vi "Configure slider scale.vi"(8 "error in (no error)":errorcluster, 10 "Slide Parameters":T1, 11 "Slide in":refnum<vi>) -> (0 "error out":errorcluster, 3 "Slide reference out":refnum<vi>)   [LabVIEW 2013]
uses:
  Support/Slide Parameters.ctl
  Support/PWM Object Parameters.ctl
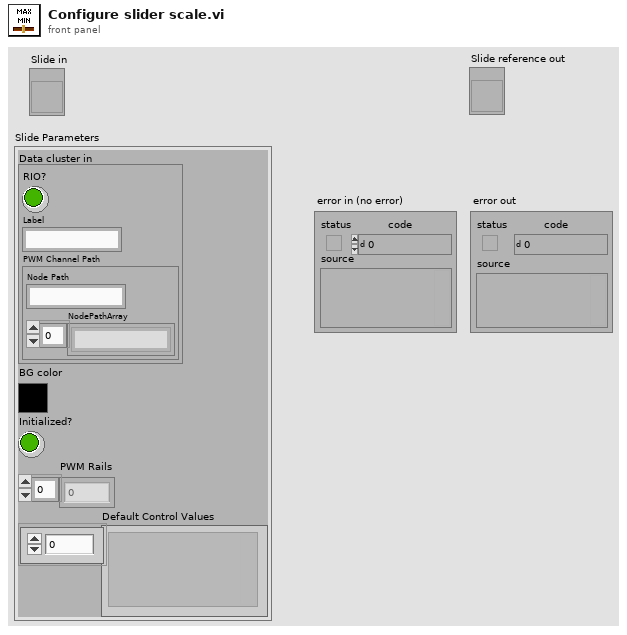
[diagram p1: front panel]
types:
  T1 = typedef "Slide Parameters.ctl" = cluster{"Data cluster in":T2, "BG color":u32, "Initialized?":bool, "PWM Rails":dbl[], "Default Control Values":variant[]}
  T2 = typedef "PWM Object Parameters.ctl" = cluster{"RIO?":bool, "Label":string, "PWM Channel Path":cluster{"NodePathArray":string[], "Node Path":string}}
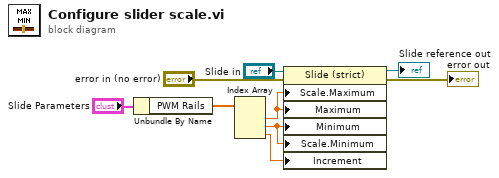
[diagram p0: block diagram]
diagram:
  n1 = Unbundle By Name("Slide Parameters") -> ("PWM Rails"=w9:dbl[])
  n2 = Index Array(array=w9) -> (element #1=w5:dbl, element #2=w4:dbl, element #3=w6:dbl)  [unwired: 3 in]
  n3 = property class="Slide (strict)"(reference="Slide in", error in="error in (no error)", "Scale.Maximum"=w5, "Maximum"=w5, "Minimum"=w4, "Scale.Minimum"=w4, "Increment"=w6) -> (reference out=→"Slide reference out":refnum<vi>, error out=→"error out":errorcluster)
